vi "Create From Euler Angles.vi"(8 "error in":errorcluster, 9 "phi/roll":dbl, 10 "theta/pitch":dbl, 11 "psi/yaw":dbl) -> (0 "error out":errorcluster, 3 "Orient3d out":refnum<class "Orient3d Class.lvclass">)   [LabVIEW 2011, in "Orient3d Class.lvclass"]
uses:
  Orient3d Class.lvclass
  Type Definitions/Quaternion.ctl
  Orient3d Class.lvclass/Orient3d Class.ctl
panel:
  # "Uses angle conventions from\nhttps://en.wikipedia.org/wiki/Conversion_between_quaternions_and_Euler_angles"
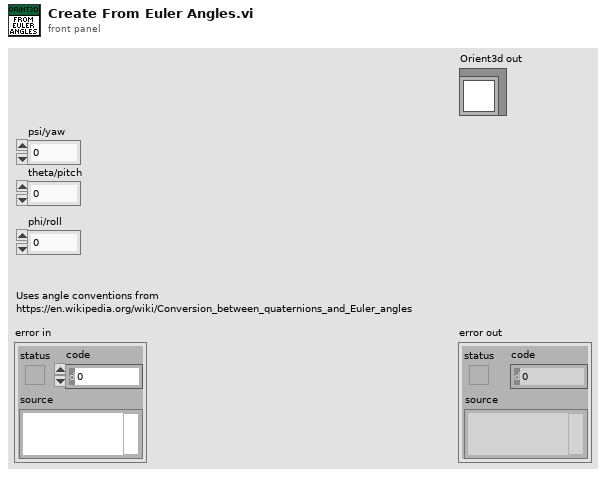
[diagram p1: front panel]
types:
  T1 = typedef "Quaternion.ctl" = cluster{"x":dbl, "y":dbl, "z":dbl, "w":dbl}
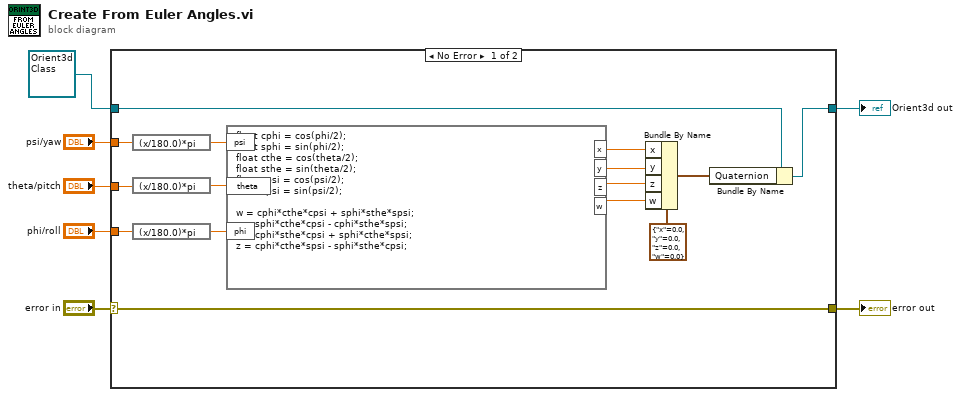
[diagram p0: block diagram]
diagram:
  n1 = case shown="No Error" "error in" {
    selector: "error in" -> [w22 w24]
    tunnel: [w22 w24] -> w6
    tunnel: [w14 w23] -> w4
    tunnel: refnum<class "Orient3d Class.lvclass"> refnum ("Orient3d Class in") -> [w16 w23]
    tunnel: "psi/yaw" -> [w13 _]
    tunnel: "theta/pitch" -> [w11 _]
    tunnel: "phi/roll" -> [w9 _]
    frame No Error {
      n2 = expression code="(x/180.0)*pi" ("degrees to radians")(w13) -> (w12:dbl)
      n3 = expression code="(x/180.0)*pi" ("degrees to radians")(w11) -> (w10:dbl)
      n4 = expression code="(x/180.0)*pi" ("degrees to radians")(w9) -> (w8:dbl)
      n5 = formula code="float cphi = cos(phi/2);\nfloat sphi = sin(phi/2);\nfloat cthe = cos(theta/2);\nfloat sthe = sin(theta/2);\nfloat cpsi = cos(psi/2);\nfloat spsi = sin(psi/2);\n\nw = cphi*cthe*cpsi + sphi*sthe*spsi;\nx = sphi*cthe*cpsi - cphi*sthe*spsi;\ny = cphi*sthe*cpsi + sphi*cthe*spsi;\nz = cphi*cthe*spsi - sphi*sthe*cpsi;"("psi"=w12, "theta"=w10, "phi"=w8) -> ("x"=w20:dbl, "y"=w19:dbl, "z"=w18:dbl, "w"=w17:dbl)
      n6 = Bundle By Name(cluster=T1 {"x"=0.0, "y"=0.0, "z"=0.0, "w"=0.0} ("Quaternion"), "x"=w20, "y"=w19, "z"=w18, "w"=w17) -> (w15:T1)
      n7 = Bundle By Name(cluster=w16, "Quaternion"=w15) -> (w14:refnum<class "Orient3d Class.lvclass">)
    }
    frame Error {
    }
  }
  "error out" <- w6
  "Orient3d out" <- w4
